vi "SLSC Write Properties.vi"(0 "session in":refnum<k21>, 1 "Stop Updating?":bool, 3 "Detect?":bool[](array[boolean]), 5 "SLSC Module Name":refnum<k21>, 9 "Values":dbl[](array[numeric]), 11 "error in":errorcluster, 12 "SLSC Dynamic Outputs":T1[](array[typedef])) -> (4 "session out":refnum<k21>, 6 "SLSC Module Name":refnum<k21>, 8 "LoopRate(ms)":u32=50, 15 "error out":errorcluster)   [LabVIEW 2017, in "SLSC CD Engine.lvlib"]
uses:
  SLSC CD Engine.lvlib
  SLSC Dynamic Channel.ctl
  SLSC Datatype.ctl
  <vilib>/SLSC/Commit Properties for Devices.vi
  <vilib>/SLSC/Set Generic Property (U64).vi
  <vilib>/SLSC/Set Generic Property (U32).vi
  <vilib>/SLSC/Set Generic Property (String).vi
  <vilib>/SLSC/Set Generic Property (I64).vi
  <vilib>/SLSC/Set Generic Property (I32).vi
  <vilib>/SLSC/Set Generic Property (DBL).vi
  <vilib>/SLSC/Set Generic Property (Bool).vi
  <vilib>/SLSC/SLSC.lvlib
  <vilib>/NI VeriStand/Custom Device Tools/Custom Device Utility Library/Custom Device Utility Library.lvlib
  SLSC CD Shared/SLSC CD Shared.lvlib
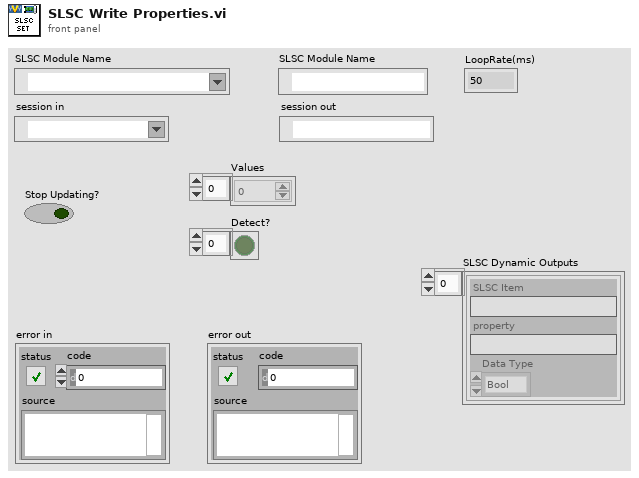
[diagram p1: front panel]
types:
  T1 = typedef "SLSC CD Shared.lvlib/SLSC Dynamic Channel.ctl" = cluster{"SLSC Item":string, "property":string, "Data Type":T2}
  T2 = typedef "SLSC CD Shared.lvlib/SLSC Datatype.ctl" = enum16{"Bool", "Double", "I32", "I64", "String", "U32", "U64"}
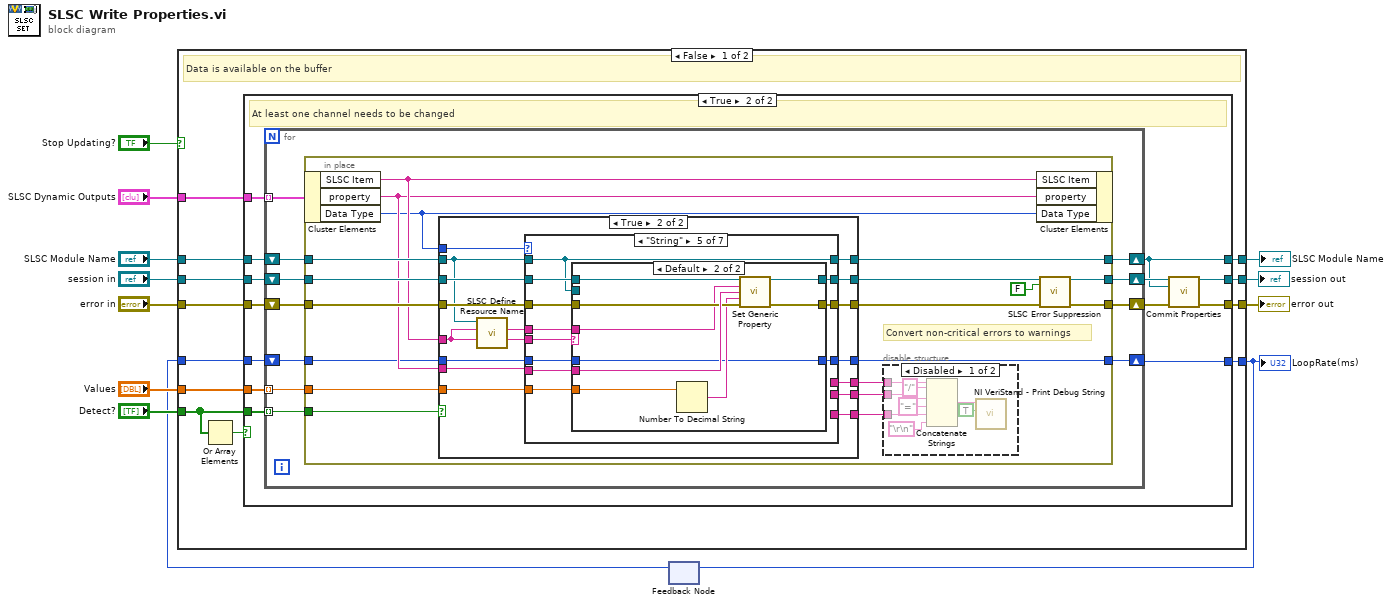
[diagram p0: block diagram]
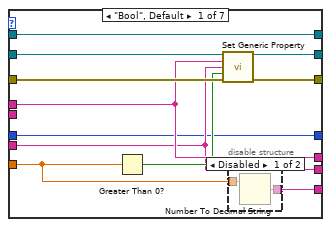
[diagram p5: hidden frame]
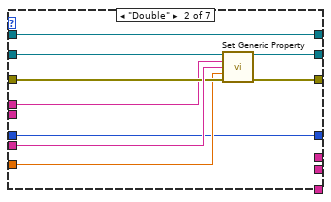
[diagram p7: hidden frame]
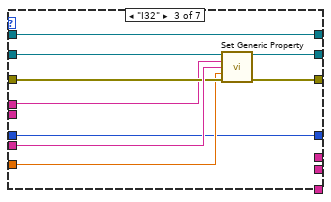
[diagram p8: hidden frame]
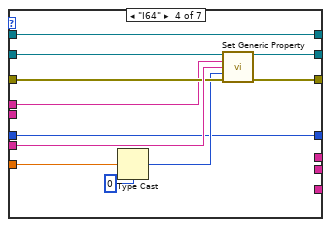
[diagram p9: hidden frame]
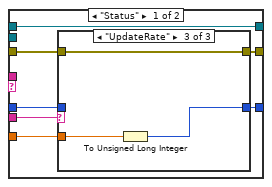
[diagram p10: hidden frame]
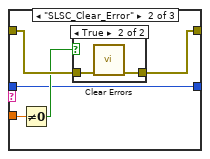
[diagram p12: hidden frame]
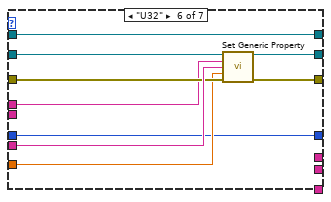
[diagram p14: hidden frame]
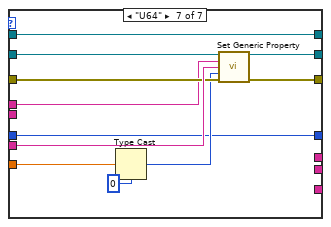
[diagram p15: hidden frame]
diagram:
  n1 = feedback #1() -> (w1:u32)  [unwired: 1 in]
  n2 = case shown="False" "Stop Updating?" {
    tunnel: "error in" -> [w24 w202]
    tunnel: "SLSC Dynamic Outputs" -> [w23 _]
    tunnel: "Values" -> [w22 _]
    tunnel: "session in" -> [w21 w203]
    tunnel: "SLSC Module Name" -> [w20 w204]
    tunnel: [w14 w204] -> w8
    tunnel: [w19 w202] -> w7
    tunnel: [w18 w203] -> w6
    tunnel: "Detect?" -> [w17 _]
    tunnel: [w15 w201] -> w2
    tunnel: w1 -> [w16 w201]
    frame False {
      # "Data is available on the buffer"
      n3 = Or Array Elements(Boolean array=w17) -> (logical OR=w13:bool)
      n4 = case shown="True" w13 {
        tunnel: w24 -> [w26 w41]
        tunnel: w23 -> [_ w40]
        tunnel: w22 -> [_ w39]
        tunnel: w21 -> [w27 w38]
        tunnel: w20 -> [w28 w37]
        tunnel: [w26 w35] -> w19
        tunnel: [w27 w33] -> w18
        tunnel: w17 -> [_ w32]
        tunnel: w16 -> [w25 w31]
        tunnel: [w25 w30] -> w15
        tunnel: [w28 w29] -> w14
        frame False {
          # "Do change detected, bypass write action"
        }
        frame True {
          # "At least one channel needs to be changed"
          n5 = for {
            tunnel: w39 -> [w52] mode=indexing
            tunnel: w40 -> [w45] mode=indexing
            shift-right: [w50] -> w34
            shift-left: w38 -> [w51]
            shift-right: [w49] -> w29
            shift-left: w37 -> [w46]
            tunnel: w32 -> [w44] mode=indexing
            shift-right: [w42] -> w30
            shift-left: w31 -> [w43]
            shift-right: [w47] -> w36
            shift-left: w41 -> [w48]
            n6 = in-place {
              in-place-border: w52 -> [w62]
              in-place-border: w51 -> [w70]
              in-place-border: [w69] -> w50
              in-place-border: [w68] -> w49
              in-place-border: w48 -> [w67]
              in-place-border: [w53] -> w47
              in-place-border: w46 -> [w66]
              in-place-border: w44 -> [w58]
              in-place-border: [w56] -> w42
              in-place-border: w43 -> [w55]
              # "Convert non-critical errors to warnings"
              n7 = in-place-cluster #2(w45) -> ("SLSC Item"=w65:string, "property"=w64:string, "Data Type"=w63:T2)
              n8 = case shown="True" w58 {
                tunnel: w70 -> [w81 w98]
                tunnel: [w81 w97] -> w69
                tunnel: [w82 w96] -> w68
                tunnel: w67 -> [w80 w95]
                tunnel: [w80 w94] -> w57
                tunnel: w66 -> [w82 w93]
                tunnel: w65 -> [_ w91]
                tunnel: w64 -> [_ w90]
                tunnel: w63 -> [_ w89]
                tunnel: w62 -> [_ w88]
                tunnel: [_ w87] -> w61
                tunnel: [_ w86] -> w60
                tunnel: [_ w85] -> w59
                tunnel: [w79 w84] -> w56
                tunnel: w55 -> [w79 w83]
                frame False {
                }
                frame True {
                  n9 = call "SLSC Define Resource Name.vi"("SLSC Item"=w91, "SLSC Module Name"=w93) -> ("Resource"=w92:string)  [unwired: 9 in]
                  n10 = case shown="\"String\"" w89 {
                    tunnel: w88 -> [w104 w114 w123 w134 w146 w183 w193]
                    tunnel: w98 -> [w109 w120 w129 w140 w151 w189 w200]
                    tunnel: [w108 w119 w128 w139 w150 w188 w199] -> w97
                    tunnel: w90 -> [w101 w118 w127 w138 w149 w187 w198]
                    tunnel: w93 -> [w107 w117 w126 w137 w145 w186 w197]
                    tunnel: [w107 w117 w126 w137 w145 w186 w197] -> w96
                    tunnel: w95 -> [w106 w116 w125 w136 w148 w185 w196]
                    tunnel: [w105 w115 w124 w135 w147 w184 w195] -> w94
                    tunnel: w92 -> [w103 w113 w122 w131 w143 w182 w191]
                    tunnel: w91 -> [_ _ _ _ w144 _ _]
                    tunnel: [w103 _ _ _ _ _ _] -> w87
                    tunnel: [w101 _ _ _ _ _ _] -> w86
                    tunnel: [w100 _ _ _ _ _ _] -> w85
                    tunnel: [w99 w112 w121 w130 w142 w181 w190] -> w84
                    tunnel: w83 -> [w99 w112 w121 w130 w141 w181 w190]
                    frame "Bool", Default {
                      n11 = Greater Than 0?(x=w104) -> (x > 0?=w102:bool)
                      n12 = call-poly <vilib>:"Set Generic Property.vi"("session in"=w109, "resources"=w103, "property"=w101, "property value"=w102, "error in (no error)"=w106) -> ("session out"=w108:refnum<k21>, "error out"=w105:errorcluster)  [unwired: 9 in]
                      n13 = disable-structure shown="Disabled" {
                        disable-tunnel: w104 -> [w111 _]
                        disable-tunnel: [w110 _] -> w100
                        frame Disabled {
                          n14 = Number To Decimal String(number=w111) -> (decimal integer string=w110:string)  [unwired: 1 in]
                        }
                        frame Enabled {
                        }
                      }
                    }
                    frame "Double" {
                      n15 = call-poly <vilib>:"Set Generic Property.vi"("session in"=w120, "resources"=w113, "property"=w118, "property value"=w114, "error in (no error)"=w116) -> ("session out"=w119:refnum<k21>, "error out"=w115:errorcluster)  [unwired: 9 in]
                    }
                    frame "I32" {
                      n16 = call-poly <vilib>:"Set Generic Property.vi"("session in"=w129, "resources"=w122, "property"=w127, "property value"=w123, "error in (no error)"=w125) -> ("session out"=w128:refnum<k21>, "error out"=w124:errorcluster)  [unwired: 9 in]
                    }
                    frame "I64" {
                      n17 = Type Cast(type=i64 0 ("property value"), x=w134) -> (*(type *) &x=w132:i64)
                      n18 = call-poly <vilib>:"Set Generic Property.vi"("session in"=w140, "resources"=w131, "property"=w138, "property value"=w132, "error in (no error)"=w136) -> ("session out"=w139:refnum<k21>, "error out"=w135:errorcluster)  [unwired: 9 in]
                    }
                    frame "String" {
                      n19 = case shown="Default" w144 {
                        tunnel: w151 -> [w158 w180]
                        tunnel: [w158 w179] -> w150
                        tunnel: w149 -> [w156 w178]
                        tunnel: w145 -> [_ _]
                        tunnel: w148 -> [w154 w177]
                        tunnel: [w155 w176] -> w147
                        tunnel: w146 -> [w157 w175]
                        tunnel: w143 -> [_ w173]
                        tunnel: [w153 w172] -> w142
                        tunnel: w141 -> [w152 w172]
                        frame "Status" {
                          n20 = case shown="\"UpdateRate\"" w156 {
                            tunnel: w157 -> [_ w163 w170]
                            tunnel: [w160 w164 w171] -> w155
                            tunnel: w154 -> [w160 w165 w171]
                            tunnel: [w159 w161 w169] -> w153
                            tunnel: w152 -> [w159 w161 _]
                            frame Default {
                            }
                            frame "SLSC_Clear_Error" {
                              n21 = Not Equal To 0?(x=w163) -> (x != 0?=w162:bool)
                              n22 = case shown="True" w162 {
                                tunnel: w165 -> [w166 w168]
                                tunnel: [w166 w167] -> w164
                                frame False {
                                }
                                frame True {
                                n23 = call <vilib>:"Clear Errors.vi"("error in (no error)"=w168) -> ("error out"=w167:errorcluster)  [unwired: 5 in, 1 out]
                                }
                              }
                            }
                            frame "UpdateRate" {
                              n24 = To Unsigned Long Integer(number=w170) -> (unsigned 32bit integer=w169:u32)
                            }
                          }
                        }
                        frame Default {
                          n25 = Number To Decimal String(number=w175) -> (decimal integer string=w174:string)  [unwired: 1 in]
                          n26 = call-poly <vilib>:"Set Generic Property.vi"("session in"=w180, "resources"=w173, "property"=w178, "property value"=w174, "error in (no error)"=w177) -> ("session out"=w179:refnum<k21>, "error out"=w176:errorcluster)  [unwired: 9 in]
                        }
                      }
                    }
                    frame "U32" {
                      n27 = call-poly <vilib>:"Set Generic Property.vi"("session in"=w189, "resources"=w182, "property"=w187, "property value"=w183, "error in (no error)"=w185) -> ("session out"=w188:refnum<k21>, "error out"=w184:errorcluster)  [unwired: 9 in]
                    }
                    frame "U64" {
                      n28 = Type Cast(type=u64 0 ("property value"), x=w193) -> (*(type *) &x=w192:u64)
                      n29 = call-poly <vilib>:"Set Generic Property.vi"("session in"=w200, "resources"=w191, "property"=w198, "property value"=w192, "error in (no error)"=w196) -> ("session out"=w199:refnum<k21>, "error out"=w195:errorcluster)  [unwired: 9 in]
                    }
                  }
                }
              }
              n30 = disable-structure shown="Disabled" {
                disable-tunnel: w60 -> [w73 _]
                disable-tunnel: w59 -> [w72 _]
                disable-tunnel: w61 -> [w71 _]
                frame Disabled {
                  n31 = Concatenate Strings(w71, "/" ("string"), w73, "=" ("string"), w72, "\r\n") -> (w77:string)
                  n32 = call <vilib>:"NI VeriStand - Print Debug String.vi"("Add to log file? (T)"=TRUE, "Message"=w77) -> ()  [unwired: 9 in, 1 out]
                }
                frame Enabled {
                }
              }
              n33 = in-place-cluster #2("SLSC Item"=w65, "property"=w64, "Data Type"=w63) -> ()  [unwired: 1 out]
              n34 = call "SLSC Error Suppression.vi"("error in (no error)"=w57, "Popup Error?"=FALSE) -> ("error out"=w53:errorcluster)  [unwired: 7 in, 1 out]
            }
          }
          n35 = call-poly <vilib>:"Commit Properties.vi"("session in"=w34, "devices"=w29, "error in (no error)"=w36) -> ("session out"=w33:refnum<k21>, "error out"=w35:errorcluster)  [unwired: 11 in]
        }
      }
    }
    frame True {
      # "No data on the buffer"
    }
  }
  "error out" <- w7
  "session out" <- w6
  "SLSC Module Name" <- w8
  "LoopRate(ms)" <- w2
  n36 = feedback-in #1(w2) -> ()
